vi "Format Displays.vi"() -> (0 "cryogenlvls":cluster{"tankHe":dbl, "tankN":dbl} {"tankN" min=-1.0 max=100.0 scale=0.0..100.0; "tankHe" min=-1.0 max=100.0 scale=0.0..100.0}, 1 "tempdisp":string, 2 "ratedisp":string, 3 "fielddisp":string, 4 "per?":bool)   [LabVIEW 2009, in "Magnet.lvclass"]
uses:
  Magnet.lvclass
panel:
  # "Cryogen Levels"
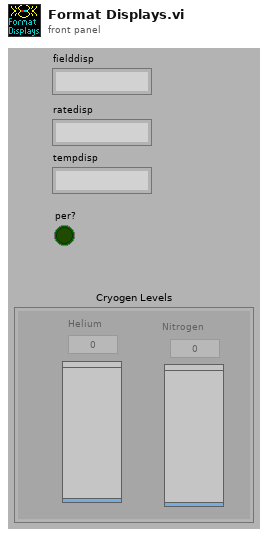
[diagram p1: front panel]
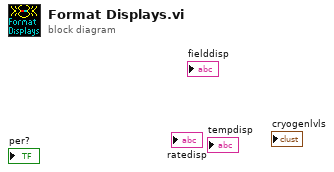
[diagram p0: block diagram]
diagram:
